vi "Photon Counter Start.vi"(0 "VISA resource name":refnum<visa-resource-name>="GPIB0::23::INSTR", 1 "Dwell Time":dbl[unit]=0.5 min=0.0 max=60.0 step=0.002 format="%#_13g", 2 "Disc A Mode":T1, 3 "Count A Input":enum16{"10 MHz", "INPUT 1", "INPUT 2", "TRIG"}(ring)=enum."INPUT 1", 4 "Count B Input":enum16{"10 MHz", "INPUT 1", "INPUT 2", "TRIG"}(ring)=enum."INPUT 1", 5 "Trigger Level":dbl=1.25 format="%#_13g", 6 "Disc B Mode":T1, 7 "errorIN":errorcluster caption="Error In", 8 "Display Mode":enum16{"Continuous", "Hold"}(ring), 9 "Count Mode":T3(ring), 11 "Trigger Slope":enum16{"Rise", "Fall"}(ring), 12 "Disc A Lvl":dbl=-0.034 format="%#_13g", 13 "# of periods":i32=3 min=0 max=2000 step=1, 14 "Disc B Lvl":dbl=-0.034 format="%#_13g", 15 "Scan End Mode":enum16{"Stop", "Start"}(ring), 16 "Count Time Set":dbl[unit]=1.0, 17 "Gate A Delay (def: 0 s)":dbl[unit]=5e-09, 18 "Gate B Delay (def: 0 s)":dbl[unit]=5e-09, 19 "Disc A\nSlope":enum16{"Rise", "Fall"}(ring), 21 "Gate A Width (def: 0 s)":dbl[unit]=5e-09, 23 "Gate B Width (def: 0 s)":dbl[unit]=5e-09, 24 "Gate B Mode":T2, 25 "Gate A Mode":T2, 26 "Disc B\nSlope":enum16{"Rise", "Fall"}(ring)) -> (20 "VISA resource name out":refnum<visa-resource-name>="GPIB0::23::INSTR", 27 "errorOUT":errorcluster caption="Error Out")   [LabVIEW 2015, in "SR400.lvlib"]
uses:
  SR400.lvlib
  Typedefs/Gate Mode.ctl
  Typedefs/Discriminator Output.ctl
  Typedefs/Counter.ctl
  Typedefs/Gate.ctl
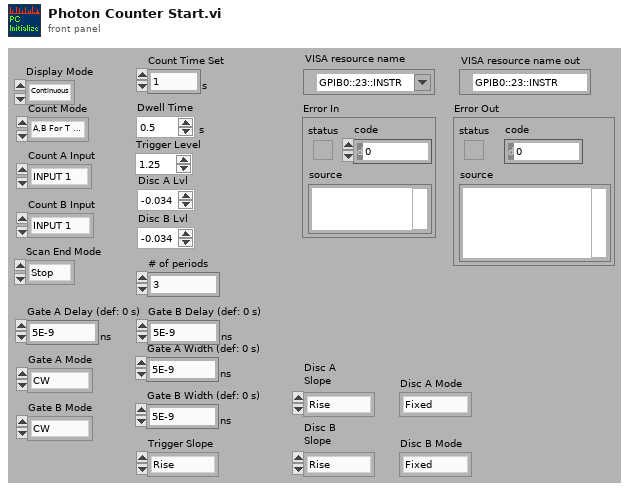
[diagram p1: front panel]
types:
  T1 = typedef "SR400.lvlib/Discriminator Output.ctl" = enum16{"Fixed", "Scan"}
  T2 = typedef "SR400.lvlib/Gate Mode.ctl" = enum16{"CW", "Fixed", "Scan"}
  T3 = enum16{"A,B For T Preset", "A-B For T Preset", "A+B For T Preset", "A For B Preset"}
  T4 = typedef "SR400.lvlib/Counter.ctl" = enum16{"Counter A", "Counter B", "Counter T"}
  T5 = typedef "SR400.lvlib/Gate.ctl" = enum16{"Gate A", "Gate B"}
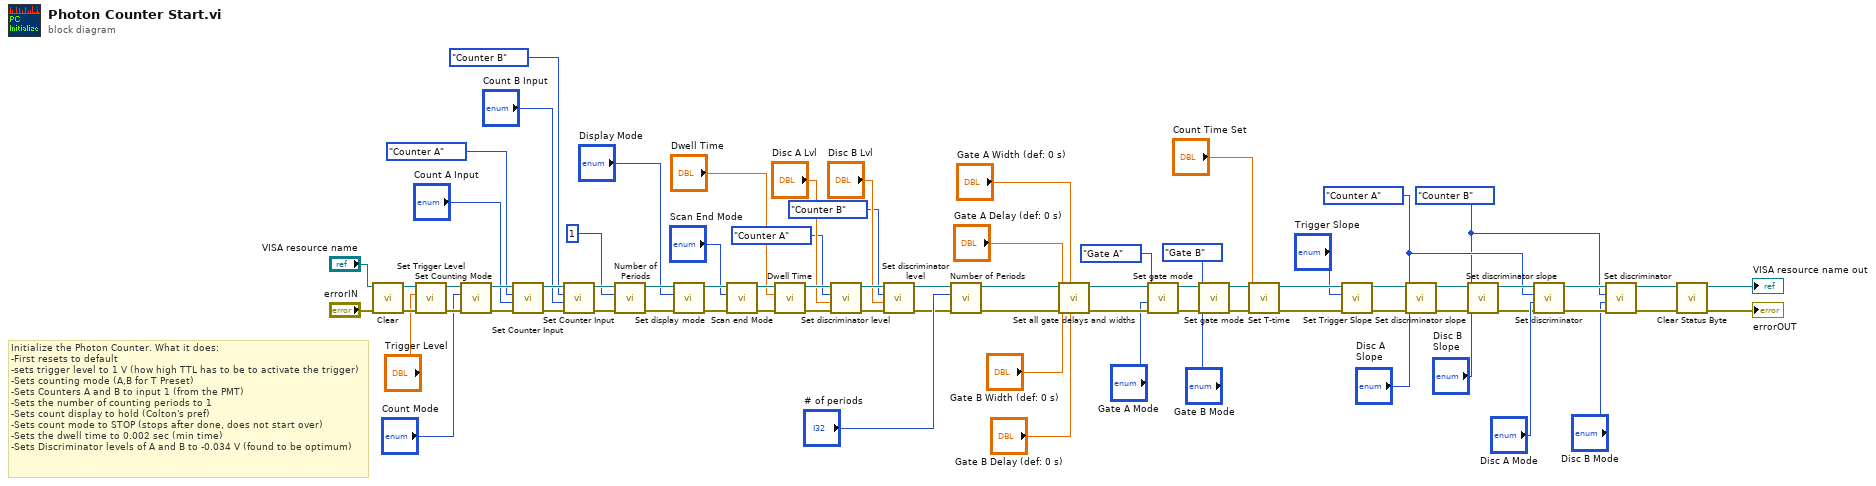
[diagram p0: block diagram]
diagram:
  w6 = Counter."Counter B" ("i (0)")
  w11 = Counter."Counter A" ("i (0)")
  # "Initialize the Photon Counter. What it does:\n-First resets to default\n-sets trigger level to 1 V (how high TTL has to be to activate the trigger) \n-Sets counting mode (A,B for T Preset)\n-Sets Counters A and B to input 1 (from the PMT)\n-Sets the number of counting periods to 1\n-Sets count display to hold (Colton's pref)\n-Sets count mode to STOP (stops after done, does not start over)\n-Sets the dwell time to 0.002 sec (min time)\n-Sets Discriminator levels of A and B to -0.034 V (found to be optimum)"
  n1 = call "Clear.vi"("error in (no error)"="errorIN", "VISA resource name"="VISA resource name") -> ("error out"=w76:errorcluster, "VISA resource name out"=w77:refnum<visa-resource-name>)  [unwired: 8 out]
  n2 = call "Set Trigger Level.vi"("error in (no error)"=w76, "Trigger Level (1 V)"="Trigger Level", "VISA resource name"=w77) -> ("error out"=w74:errorcluster, "VISA resource name out"=w75:refnum<visa-resource-name>)  [unwired: 7 out]
  n3 = call "Set Counting Mode.vi"("error in (no error)"=w74, "Mode (def: A,B for T preset)"="Count Mode", "VISA resource name"=w75) -> ("error out"=w72:errorcluster, "VISA resource name out"=w73:refnum<visa-resource-name>)  [unwired: 7 out]
  n4 = call "Set Counter Input.vi"("error in (no error)"=w72, "Input (def: 10 MHz)"="Count A Input", "Counter (def: A)"=enum16{"Counter A", "Counter B", "Counter T"}."Counter A" ("Count A Input"), "VISA resource name"=w73) -> ("error out"=w70:errorcluster, "VISA resource name out"=w71:refnum<visa-resource-name>)  [unwired: 6 out]
  n5 = call "Set Counter Input.vi"("error in (no error)"=w70, "Input (def: 10 MHz)"="Count B Input", "Counter (def: A)"=enum16{"Counter A", "Counter B", "Counter T"}."Counter B" ("Count B Input"), "VISA resource name"=w71) -> ("error out"=w58:errorcluster, "VISA resource name out"=w59:refnum<visa-resource-name>)  [unwired: 6 out]
  n6 = call "Number of Periods.vi"("error in (no error)"=w58, "# of periods (def: 1)"=1 ("# Periods"), "VISA resource name"=w59) -> ("error out"=w68:errorcluster, "VISA resource name out"=w69:refnum<visa-resource-name>)  [unwired: 7 out]
  n7 = call "Set display mode.vi"("error in (no error)"=w68, "Display Mode (def: Hold)"="Display Mode", "VISA resource name"=w69) -> ("error out"=w66:errorcluster, "VISA resource name out"=w67:refnum<visa-resource-name>)  [unwired: 7 out]
  n8 = call "Scan end Mode.vi"("error in (no error)"=w66, "Scan End Mode (Def: Stop)"="Scan End Mode", "VISA resource name"=w67) -> ("error out"=w64:errorcluster, "VISA resource name out"=w65:refnum<visa-resource-name>)  [unwired: 7 out]
  n9 = call "Dwell Time.vi"("error in (no error)"=w64, "Dwell time (0.002 s)"="Dwell Time", "VISA resource name"=w65) -> ("error out"=w62:errorcluster, "VISA resource name out"=w63:refnum<visa-resource-name>)  [unwired: 7 out]
  n10 = call "Set discriminator level.vi"("error in (no error)"=w62, "Level (-0.034 V)"="Disc A Lvl", "Discriminator (def: A)"=Counter."Counter A", "VISA resource name"=w63) -> ("error out"=w60:errorcluster, "VISA resource name out"=w61:refnum<visa-resource-name>)  [unwired: 6 out]
  n11 = call "Set discriminator level.vi"("error in (no error)"=w60, "Level (-0.034 V)"="Disc B Lvl", "Discriminator (def: A)"=Counter."Counter B", "VISA resource name"=w61) -> ("error out"=w39:errorcluster, "VISA resource name out"=w40:refnum<visa-resource-name>)  [unwired: 6 out]
  n12 = call "Number of Periods.vi"("error in (no error)"=w39, "# of periods (def: 1)"="# of periods", "VISA resource name"=w40) -> ("error out"=w37:errorcluster, "VISA resource name out"=w38:refnum<visa-resource-name>)  [unwired: 7 in]
  n13 = call "Set all gate delays and widths.vi"("Gate B Delay (def: 0 s)"="Gate B Delay (def: 0 s)", "Gate A Width (def: 0 s)"="Gate A Width (def: 0 s)", "error in (no error)"=w37, "Gate B Width (def: 0 s)"="Gate B Width (def: 0 s)", "Gate A Delay (def: 0 s)"="Gate A Delay (def: 0 s)", "VISA resource name"=w38) -> ("error out"=w31:errorcluster, "VISA resource name out"=w32:refnum<visa-resource-name>)  [unwired: 4 in]
  n14 = call "Set gate mode.vi"("error in (no error)"=w31, "Mode (def: CW)"="Gate A Mode", "Gate (def: A)"=Gate."Gate A", "VISA resource name"=w32) -> ("error out"=w25:errorcluster, "VISA resource name out"=w27:refnum<visa-resource-name>)  [unwired: 6 in]
  n15 = call "Set gate mode.vi"("error in (no error)"=w25, "Mode (def: CW)"="Gate B Mode", "Gate (def: A)"=Gate."Gate B", "VISA resource name"=w27) -> ("error out"=w24:errorcluster, "VISA resource name out"=w26:refnum<visa-resource-name>)  [unwired: 6 in]
  n16 = call "Set T-time.vi"("errorIN"=w24, "Count Time Set"="Count Time Set", "VISA resource name"=w26) -> ("errorOUT"=w21:errorcluster, "VISA resource name out"=w20:refnum<visa-resource-name>)  [unwired: 4 in, 1 out]
  n17 = call "Set Trigger Slope.vi"("error in (no error)"=w21, "j (0)"="Trigger Slope", "VISA resource name"=w20) -> ("error out"=w17:errorcluster, "VISA resource name out"=w18:refnum<visa-resource-name>)  [unwired: 7 in]
  n18 = call "Set discriminator slope.vi"("error in (no error)"=w17, "j (0)"="Disc A\nSlope", "i (0)"=w11, "VISA resource name"=w18) -> ("error out"=w14:errorcluster, "VISA resource name out"=w15:refnum<visa-resource-name>)  [unwired: 6 in]
  n19 = call "Set discriminator slope.vi"("error in (no error)"=w14, "j (0)"="Disc B\nSlope", "i (0)"=w6, "VISA resource name"=w15) -> ("error out"=w9:errorcluster, "VISA resource name out"=w12:refnum<visa-resource-name>)  [unwired: 6 in]
  n20 = call "Set discriminator.vi"("error in (no error)"=w9, "j (0)"="Disc A Mode", "i (0)"=w11, "VISA resource name"=w12) -> ("error out"=w7:errorcluster, "VISA resource name out"=w8:refnum<visa-resource-name>)  [unwired: 6 in]
  n21 = call "Set discriminator.vi"("error in (no error)"=w7, "j (0)"="Disc B Mode", "i (0)"=w6, "VISA resource name"=w8) -> ("error out"=w4:errorcluster, "VISA resource name out"=w3:refnum<visa-resource-name>)  [unwired: 6 in]
  n22 = call "Clear Status Byte.vi"("error in (no error)"=w4, "VISA resource name"=w3) -> ("error out"=→"errorOUT":errorcluster, "VISA resource name out"=→"VISA resource name out":refnum<visa-resource-name>)  [unwired: 8 in]
